vi "Show Panel.vi"(8 "error in (no error)":errorcluster, 10 "Open Diagram Argument":T1) -> (0 "error out":errorcluster)   [LabVIEW 2020, in "Peek Window.lvlib"]
doc: "Send the Show Panel request to the Module's Main.vi.\n_____\nBased on Delacor QMH Project Template 5.0.0.82."
uses:
  Peek Window.lvlib
  Open Diagram Argument--cluster.ctl
  VI Types/Standard VI Type/Standard VI Type.lvclass
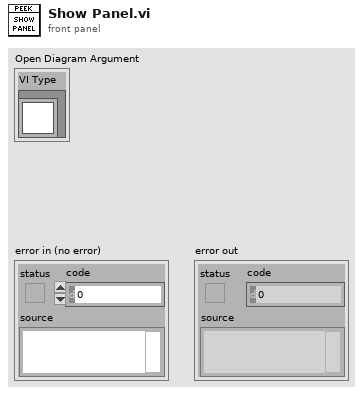
[diagram p1: front panel]
types:
  T1 = typedef "Peek Window.lvlib/Open Diagram Argument--cluster.ctl" = cluster{"VI Type":refnum<class "Standard VI Type.lvclass">}
  T2 = typedef "Peek Window.lvlib/Request Events--cluster.ctl" = cluster{"Stop Module":refnum<user-event>, "Show Panel":refnum<user-event>, "Hide Panel":refnum<user-event>, "Get Module Execution Status":refnum<user-event>, "Show Diagram":refnum<user-event>, "Open Diagram":refnum<user-event>, "Invalid Selection":refnum<user-event>}
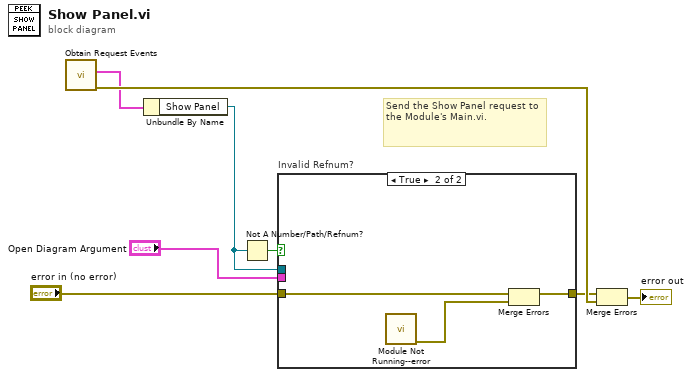
[diagram p0: block diagram]
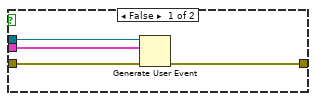
[diagram p2: hidden frame]
diagram:
  # "Send the Show Panel request to the Module's Main.vi."
  n1 = call "Obtain Request Events.vi"() -> ("error out"=w7:errorcluster, "Peek Window Request Events"=w6:T2)  [unwired: 10 in]
  n2 = Unbundle By Name(w6) -> ("Show Panel"=w4:refnum<user-event>)
  n3 = Not A Number/Path/Refnum?(number/path/refnum=w4) -> (NaN/Path/Refnum?=w5:bool)
  n4 = case "Invalid Refnum?" shown="True" w5 {
    tunnel: "error in (no error)" -> [w12 w15]
    tunnel: [w11 w14] -> w2
    tunnel: w4 -> [w10 _]
    tunnel: "Open Diagram Argument" -> [w9 _]
    frame False {
      n5 = Generate User Event(user event=w10, event data cluster=w9, error in=w12) -> (error out=w11:errorcluster)  [unwired: 1 in, 1 out]
    }
    frame True {
      n6 = call "Module Not Running--error.vi"() -> ("error out"=w13:errorcluster)  [unwired: 11 in]
      n7 = Merge Errors(w15, w13) -> (w14:errorcluster)
    }
  }
  n8 = Merge Errors(w2, w7) -> (→"error out":errorcluster)
